vi "StartDIDs.vi"(8 "error in (no error)":errorcluster, 11 "Connection Info":T1) -> (0 "error out":errorcluster, 3 "Connection Info":T1)   [LabVIEW 2013, in "Diagnostics Host Automation API.lvlib"]
uses:
  Diagnostics Host Automation API.lvlib
  <userlib>/STM/TCP/stm_TCP Connection Info.ctl
  <userlib>/STM/_SubVIs/stm_MetaDataElement.ctl
  <userlib>/STM/TCP/STM Write Message (TCP).vi
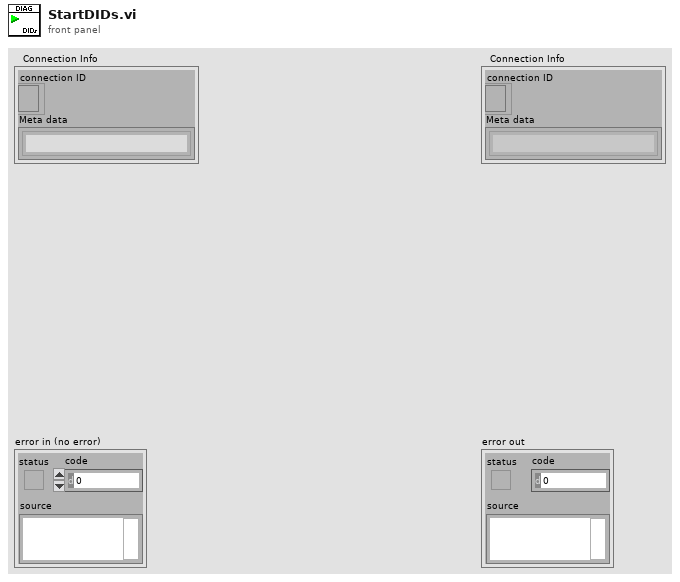
[diagram p1: front panel]
types:
  T1 = typedef "stm_TCP Connection Info.ctl" = cluster{"connection ID":refnum<k5>, "Meta data":T2[]}
  T2 = typedef "stm_MetaDataElement.ctl" = string
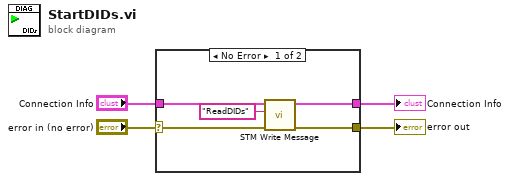
[diagram p0: block diagram]
diagram:
  n1 = case shown="No Error" "error in (no error)" {
    selector: "error in (no error)" -> [w5 w11]
    tunnel: "Connection Info" -> [w9 w10]
    tunnel: [w8 w10] -> w3
    tunnel: [w7 w11] -> w2
    frame No Error {
      n2 = call-poly <userlib>:"STM Write Message.vi"("error in (no error)"=w5, "Name"="ReadDIDs", "Connection Info"=w9) -> ("error out"=w7:errorcluster, "Connection Info Out"=w8:T1)  [unwired: 7 in]
    }
    frame Error {
    }
  }
  "Connection Info" <- w3
  "error out" <- w2
